vi "Layer Scan V6.vi"() -> ()   [LabVIEW 2025]
uses:
  <vilib>/DAQmx/write.llb/DAQmx Write (Analog 1D DBL NChan 1Samp).vi
  <vilib>/DAQmx/create/channels.llb/DAQmx Create Channel (AO-Voltage-Basic).vi
  <vilib>/DAQmx/miscellaneous.llb/DAQmx Fill In Error Info.vi
  <instrlib>/niScope/Configure/Trigger/niScope Configure Trigger Edge.vi
  <instrlib>/niScope/Configure/Trigger/niScope Configure Trigger Immediate.vi
  <instrlib>/niScope/Acquire/Fetch/niScope Multi Fetch.vi
panel:
  in  "Digitizer Channel":string
  in  "Min Record Length":i32=1000
  out "Waveform Graph 2":dbl[](graph) caption="averaged wfm"
  in  "Enforce Realtime":bool=TRUE
  out "Waveform Graph":dbl[][](graph)
  in  "Min. Sample Rate":dbl=1000000.0 format="%#_6p"
  in  "Trigger Type":u16(ring) items=["Edge", "Immediate"]
  in  "Timeout (s)":dbl=5.0 caption="Timeout(s)" format="%.2f"
  in  "Coupling":u16(ring)=1 caption="Trigger Coupling" items=["AC"=0, "DC"=1, "HF Reject"=3, "LF Reject"=4, "AC Plus HF Reject"=1001]
  in  "Trigger Source":string(combo)="0"
  in  "Stop Button":bool
  in  "Vertical Coupling":i32(ring)=1 items=["AC", "DC", "Ground"]
  in  "Num. averages":i32=64
  in  "Resource Name":refnum<k15>="Dev1" caption="Resource Name(s)"
  in  "Simulate?":bool
  out "decimated array 2":dbl[](array[numeric])
  out "decimated array":dbl[](array[numeric])
  out "Y coord filename":i32
  out "x coord file name":i32
  out "Filename Out":path
  in  "Data File Name":path
  in  "Data folder Path":path
  in  "X offset":dbl
  in  "Y offset":dbl
  in  "step":dbl
  in  "Y Count":dbl
  in  "X Count":dbl
  # "Channels and Destinations"
  # "CONFIGURE SCAN"
  # "Constant Parameters"
  # "offset -> dimensions\n10 mm ~= 70 units\n1.5 mm ~= 10 units"
  # "Wave Propagation and Signal Strength Scan Guide"
  # "Signal Strength Scan Only Guide"
  # "1. 'Digitizer Channel' - type in '0,1'\n\n2. 'Resource name' same as SS scan\n\n3. Define data file destination and name\n\n4. Ensure 'Trigger type is set to 'Edge' \n\n5. Choose sample rate. (MAX 2.5 Gs/s)\n\n6. X and Y count must be non-zero\n\n7. Set scan starting offset (from center)\n\n8. Select step size\n\n9. Set 'Num. Averages' to desired value (based on noise).\nWill increase time to finish scan"
  # "1. 'Digitizer Channel' - type in '1'\n\n2. 'Resource Name' - select PXI1Slot2 (visible in NI MAX)\n\n3. Copy and Paste the full path to your data folder\n\n4. Choose a name for your data files\n\n5. Ensure 'Trigger Type' is set to 'Immediate'\n\n6. Choose a sample rate (arbitrary for signal strength)\n\n7. Ensure your count for X and Y axes are NON-ZERO\n\n8. Set the scan starting point by using the 'offset' controls\n\n9. Pick your 'distance' between each point (if your offset coordinate\nstarts at the MAXIMUM coordinates, your 'step' shoud be negative).\ne.g. offset  = (700, 500), then step will have to be (-10).\n\n10. For 'Num. Averages', set to 1. (no need to average because noise isnt a factor)."
  # "General Tips"
  # "1. To have an idea of where youre scanning, play with the offsets using X and Y count == 1\nUsing the SS scan guide\n\n2. Your scan area along each axis will be equal to (X/Y count * Step). \nThe unit is Volts/100 signalled to the ."
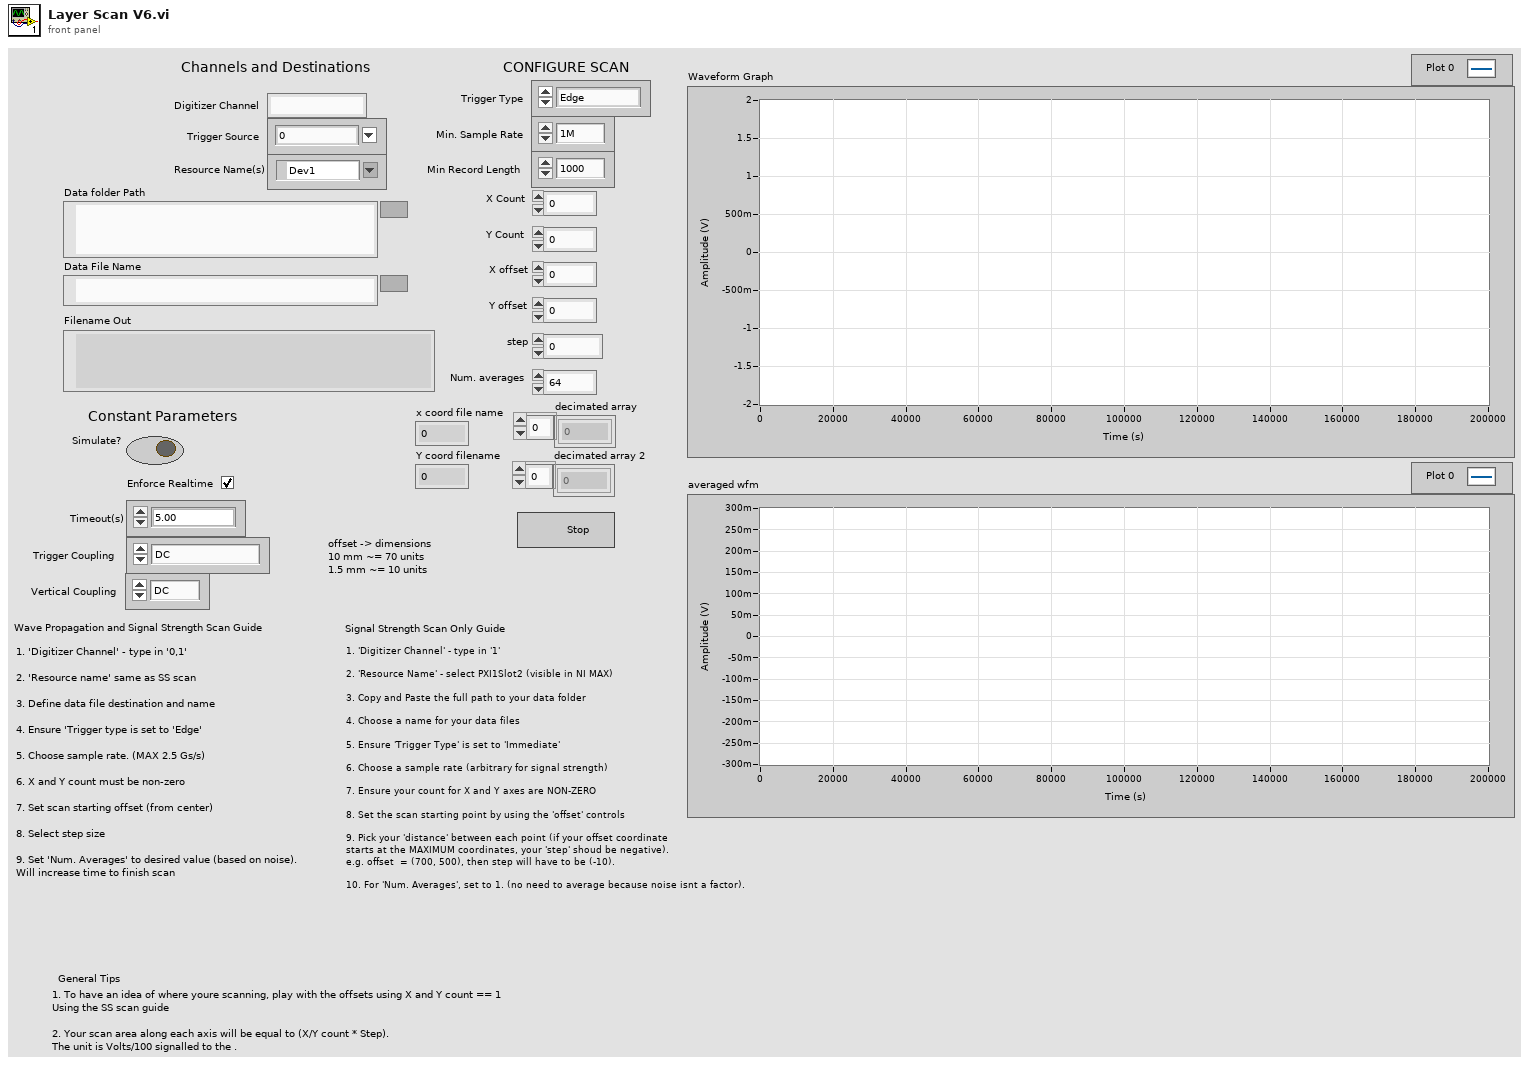
[diagram p1: front panel]
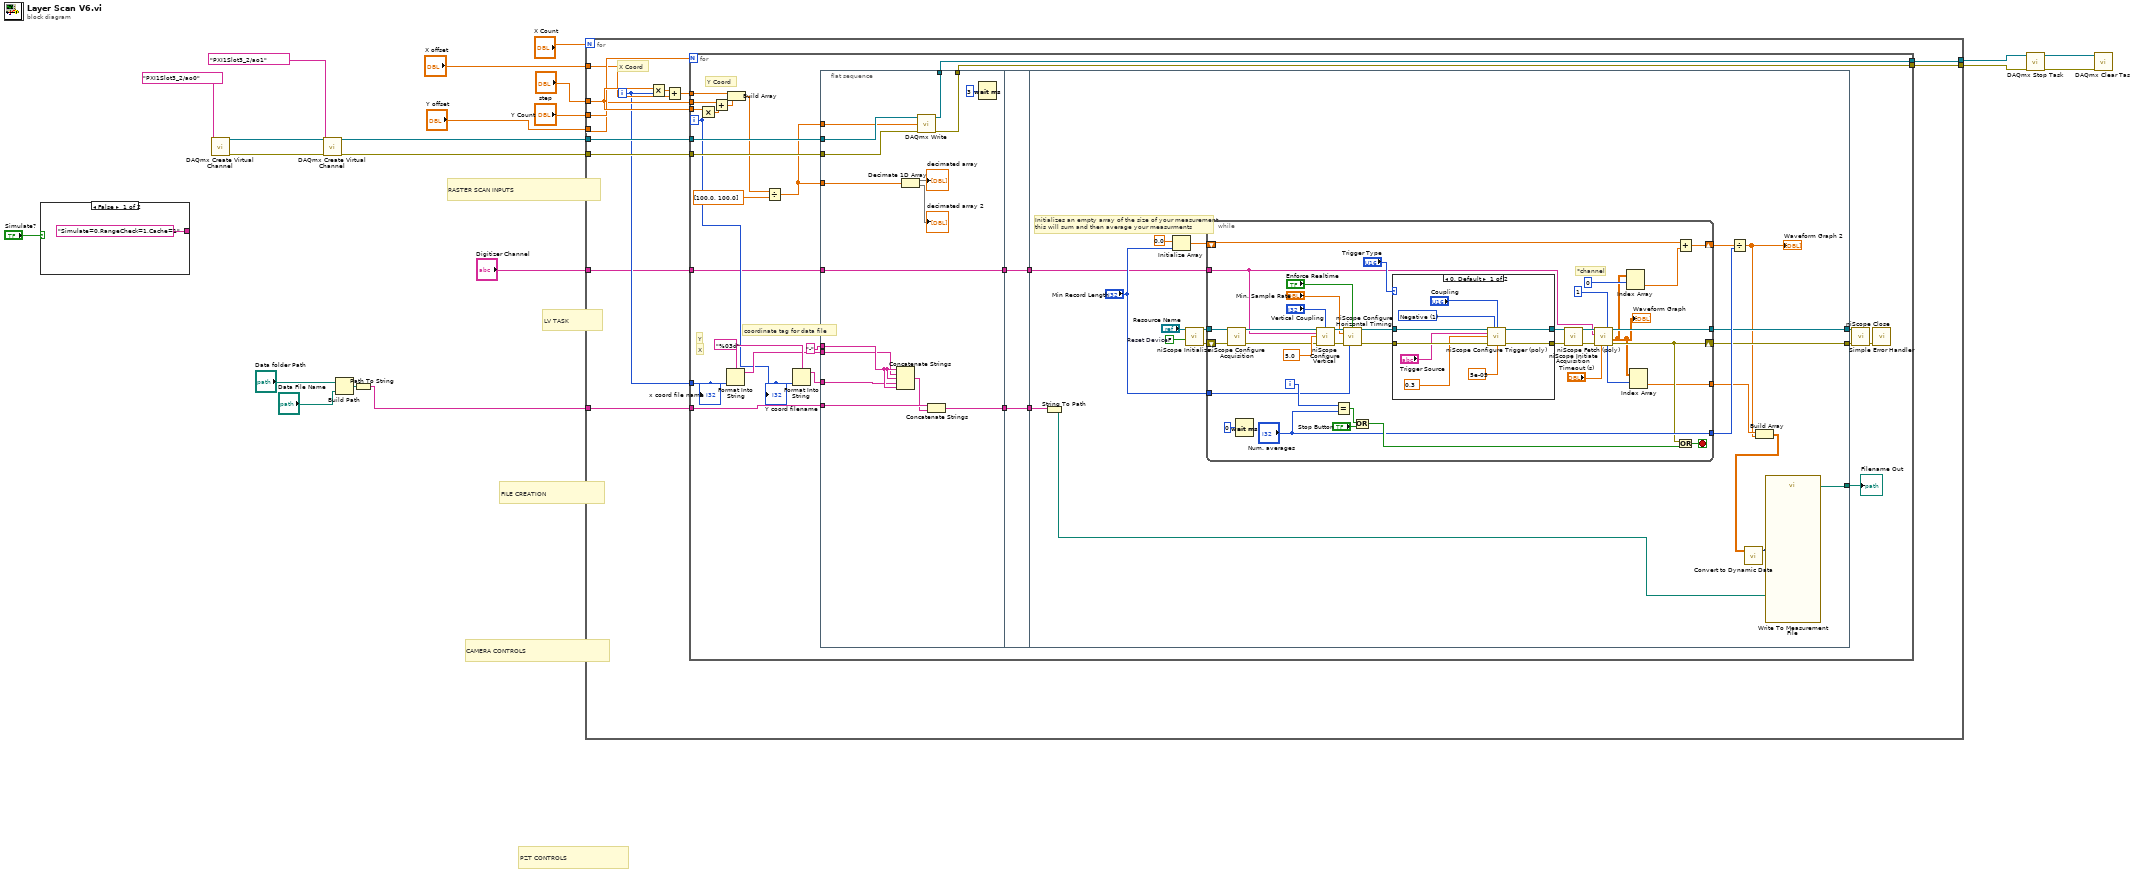
[diagram p0: block diagram]
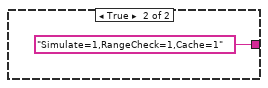
[diagram p2: hidden frame]
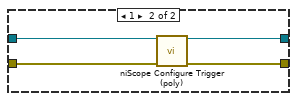
[diagram p3: hidden frame]
diagram:
  # "FILE CREATION"
  # "PZT CONTROLS"
  # "CAMERA CONTROLS"
  # "LV TASK"
  # "RASTER SCAN INPUTS"
  n1 = case shown="False" "Simulate?" {
    tunnel: ["Simulate=0,RangeCheck=1,Cache=1" ("option string") "Simulate=1,RangeCheck=1,Cache=1" ("option string")] -> _
    frame False {
    }
    frame True {
    }
  }
  n2 = call-poly <vilib>:"DAQmx Create Virtual Channel.vi"("physical channels"=tag "PXI1Slot3_2/ao0") -> ("task out"=w14:refnum<k21>, "error out"=w13:errorcluster)  [unwired: 13 in]
  n3 = call-poly <vilib>:"DAQmx Create Virtual Channel.vi"("task in"=w14, "physical channels"=tag "PXI1Slot3_2/ao1", "error in"=w13) -> ("task out"=w12:refnum<k21>, "error out"=w11:errorcluster)  [unwired: 11 in]
  n4 = Build Path(base path="Data folder Path", name or relative path="Data File Name") -> (appended path=w4:path)
  n5 = Path To String(path=w4) -> (string=w3:string)
  n6 = for {
    N: "X Count" -> [_]
    tunnel: "step" -> [w36]
    tunnel: "Y Count" -> [w35]
    tunnel: "Y offset" -> [w34]
    tunnel: "X offset" -> [w32]
    tunnel: w12 -> [w30]
    tunnel: w11 -> [w29]
    tunnel: [w28] -> w10
    tunnel: [w27] -> w9
    tunnel: w3 -> [w26]
    tunnel: "Digitizer Channel" -> [w24]
    i -> [w25]
    # "X Coord"
    n7 = Multiply(x=w36, y=w25) -> (x*y=w33:dbl)
    n8 = Add(x=w33, y=w32) -> (x+y=w31:dbl)
    n9 = for {
      N: w35 -> [_]
      tunnel: w36 -> [w64]
      tunnel: w34 -> [w62]
      tunnel: w31 -> [w61]
      tunnel: w30 -> [w59]
      tunnel: w29 -> [w58]
      tunnel: [w56] -> w28
      tunnel: [w55] -> w27
      tunnel: w26 -> [w50]
      tunnel: w25 -> [w46]
      tunnel: w24 -> [w42]
      i -> [w45]
      w54 = "%03d" ("format string")
      # "coordinate tag for data file"
      # "X"
      # "Y"
      # "Y Coord"
      n10 = Multiply(x=w64, y=w45) -> (x*y=w63:dbl)
      n11 = Add(x=w62, y=w63) -> (x+y=w60:dbl)
      n12 = Format Into String(format string=w54, w46) -> (resulting string=w52:string)  [unwired: 2 in, 1 out]
      n13 = Build Array(w61, w60) -> (w57:dbl[])
      n14 = Divide(x=w57, y=dbl[] [100.0, 100.0]) -> (x/y=w44:dbl[])
      n15 = Format Into String(format string=w54, w45) -> (resulting string=w51:string)  [unwired: 2 in, 1 out]
      n16 = flat-sequence {
        tunnel: w59 -> [w79]
        tunnel: w58 -> [w78]
        tunnel: [w77] -> w56
        tunnel: [w76] -> w55
        tunnel: "-" ("string") -> [w75]
        tunnel: w52 -> [w74]
        tunnel: w51 -> [w73]
        tunnel: w50 -> [w72]
        tunnel: [w70] -> w49
        tunnel: w44 -> [w69]
        tunnel: w44 -> [w68]
        tunnel: w42 -> [w65]
        tunnel: [w65] -> w40
        tunnel: w49 -> [w82]
        tunnel: [w82] -> w48
        tunnel: [w81] -> w41
        tunnel: w40 -> [w81]
        tunnel: w48 -> [w100]
        tunnel: [w101] -> w43
        tunnel: w41 -> [w89]
        tunnel: [w88] -> w38
        tunnel: [w87] -> w37
        frame #0 {
          n17 = Concatenate Strings(w75, w74, w75, w73, w75) -> (w71:string)
          n18 = Decimate 1D Array(w68) -> (→"decimated array":dbl[], →"decimated array 2":dbl[])
          n19 = call-poly <vilib>:"DAQmx Write.vi"("task/channels in"=w79, "data"=w69, "error in"=w78) -> ("task out"=w77:refnum<k21>, "error out"=w76:errorcluster)  [unwired: 10 in, 1 out]
          n20 = Concatenate Strings(w72, w71) -> (w70:string)
          n21 = Wait (ms)(milliseconds to wait=u32 3) -> ()  [unwired: 1 out]
        }
        frame #1 {
        }
        frame #2 {
          w98 = FALSE  # Reset Device
          # "Initializes an empty array of the size of your measurement,\nthis will sum and then average your measurments"
          n22 = String To Path(string=w100) -> (path=w99:path)
          n23 = Initialize Array(0.0 ("element"), "Min Record Length") -> (w92:dbl[])
          n24 = call <instrlib>:"niScope Initialize.vi"("resource name"="Resource Name", "reset device"=w98) -> ("instrument handle"=w96:refnum<k15>, "error out"=w95:errorcluster)  [unwired: 12 in]
          n25 = while {
            tunnel: w96 -> [w125]
            tunnel: [w109] -> w88
            shift-right: [w108] -> w87
            shift-left: w95 -> [w124]
            tunnel: ["Num. averages"] -> w94
            shift-right: [w117] -> w93
            shift-left: w92 -> [w116]
            tunnel: "Min Record Length" -> [w115]
            tunnel: w89 -> [w110]
            tunnel: [w102] -> w86
            i -> [w119]
            stop <- w126 stop-if-true
            # "*channel"
            n26 = call <instrlib>:"niScope Configure Acquisition.vi"("instrument handle"=w125, "error in"=w124) -> ("instrument handle out"=w131:refnum<k15>, "error out"=w132:errorcluster)  [unwired: 12 in]
            n27 = Wait (ms)(milliseconds to wait=u32 0 ("millisecond multiple")) -> ()  [unwired: 1 out]
            n28 = call <instrlib>:"niScope Configure Vertical.vi"("instrument handle"=w131, "vertical coupling"="Vertical Coupling", "channels"=w110, "vertical range"=5.0 ("Vertical Range (V)"), "error in"=w132) -> ("instrument handle out"=w136:refnum<k15>, "error out"=w137:errorcluster)  [unwired: 9 in]
            n29 = Equal?(x=w119, y="Num. averages") -> (x = y?=w122:bool)
            n30 = call <instrlib>:"niScope Configure Horizontal Timing.vi"("instrument handle"=w136, "enforce realtime"="Enforce Realtime", "min sample rate"="Min. Sample Rate", "error in"=w137, "min record length"=w115) -> ("instrument handle out"=w130:refnum<k15>, "error out"=w129:errorcluster)  [unwired: 9 in]
            n31 = Or(x=w122, y="Stop Button") -> (x .or. y?=w120:bool)
            n32 = case shown="0, Default" "Trigger Type" {
              tunnel: w130 -> [w146 w150]
              tunnel: w129 -> [w145 w147]
              tunnel: [w144 w149] -> w112
              tunnel: [w143 w148] -> w111
              frame 0, Default {
                w141 = u16 1 items=["Positive", "Negative"] ("Trigger Slope")
                n33 = call-poly <instrlib>:"niScope Configure Trigger (poly).vi"("instrument handle"=w146, "trigger slope"=w141, "trigger coupling"="Coupling", "trigger source"="Trigger Source", "trigger level"=0.3 ("Trigger Level"), "error in"=w145, "trigger delay"=5e-05) -> ("instrument handle out"=w144:refnum<k15>, "error out"=w143:errorcluster)  [unwired: 7 in]
              }
              frame 1 {
                n34 = call-poly <instrlib>:"niScope Configure Trigger (poly).vi"("instrument handle"=w150, "error in"=w147) -> ("instrument handle out"=w149:refnum<k15>, "error out"=w148:errorcluster)  [unwired: 12 in]
              }
            }
            n35 = call <instrlib>:"niScope Initiate Acquisition.vi"("instrument handle"=w112, "error in"=w111) -> ("instrument handle out"=w113:refnum<k15>, "error out"=w114:errorcluster)  [unwired: 12 in]
            n36 = call-poly <instrlib>:"niScope Fetch (poly).vi"("timeout"="Timeout (s)", "error in"=w114, "channels"=w110, "instrument handle"=w113) -> ("error out"=w108:errorcluster, "wfm"=w104:dbl[][], "instrument handle out"=w109:refnum<k15>)  [unwired: 4 in, 1 out]
            "Waveform Graph" <- w104
            n37 = Index Array(array=w104, index (row)=0) -> (element=w106:dbl[])  [unwired: 1 in]
            n38 = Index Array(array=w104, index (row)=1) -> (element=w102:dbl[])  [unwired: 1 in]
            n39 = Add(x=w116, y=w106) -> (x+y=w117:dbl[])
            n40 = Or(x=w108, y=w120) -> (x .or. y?=w126:bool)
          }
          n41 = Divide(x=w93, y=w94) -> (x/y=w85:dbl[])
          "Waveform Graph 2" <- w85
          n42 = Build Array(w86, w85) -> (w84:dbl[][])
          n43 = call "Convert to Dynamic Data"("2D Array"=w84) -> ("Dynamic Data Type"=w83:dynamicdata)  [unwired: 3 in]
          n44 = call "Write To Measurement File"("Signals"=w83, "Filename"=w99) -> ("Filename Out"=w101:path)  [unwired: 15 in, 2 out]
        }
      }
      n45 = call <instrlib>:"niScope Close.vi"("instrument handle"=w38, "error in"=w37) -> ("error out"=w39:errorcluster)  [unwired: 13 in]
      n46 = call <vilib>:"Simple Error Handler.vi"("error in (no error)"=w39) -> ()  [unwired: 4 in, 5 out]
      "Filename Out" <- w43
      "x coord file name" <- w46
      "Y coord filename" <- w45
    }
  }
  n47 = call <vilib>:"DAQmx Stop Task.vi"("task/channels in"=w10, "error in"=w9) -> ("task out"=w8:refnum<k21>, "error out"=w7:errorcluster)  [unwired: 12 in]
  n48 = call <vilib>:"DAQmx Clear Task.vi"("task in"=w8, "error in"=w7) -> ()  [unwired: 13 in, 1 out]
